vi "xijk_percentage_slider.vi"(8 "queue size in":i32, 9 "queue size in 2":i32, 11 "queue size max":i32) -> (0 "percentage finished":dbl, 1 "not ready?":bool, 3 "queue size out":i32)   [LabVIEW 2009]
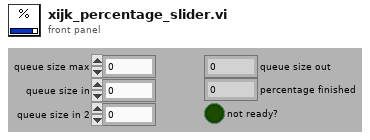
[diagram p1: front panel]
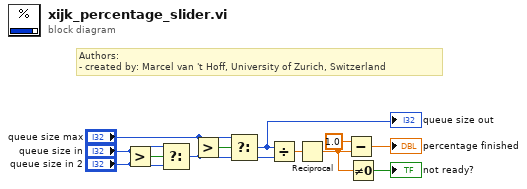
[diagram p0: block diagram]
diagram:
  # "Authors: \n- created by: Marcel van 't Hoff, University of Zurich, Switzerland"
  n1 = Greater?(x="queue size in", y="queue size in 2") -> (0:w6:bool)
  n2 = Select(t="queue size in", s=w6, f="queue size in 2") -> (s? t:f=w3:i32)
  n3 = Greater?(x="queue size max", y=w3) -> (0:w11:bool)
  n4 = Select(t="queue size max", s=w11, f=w3) -> (s? t:f=w9:i32)
  "queue size out" <- w9
  n5 = Divide(x=w9, y=w3) -> (x/y=w12:dbl)
  n6 = Reciprocal(x=w12) -> (1/x=w2:dbl)
  n7 = Subtract(x=1.0, y=w2) -> (x-y=→"percentage finished":dbl)
  n8 = Not Equal To 0?(x=w2) -> (x != 0?=→"not ready?":bool)
